vi "ModeMgr.List Modes.vi"(11 "Modes":T1[](array[typedef])=[{"Name"="", "Color"=0, "Options"=[{"Option"="Display Result Data Details", "Level"=0}, {"Option"="Not Reset SN between Tests", "Level"=0}, {"Option"="Not Validate Operator", "Level"=0}, {"Option"="Not Validate SN", "Level"=0}, {"Option"="Disable Results", "Level"=0}, {"Option"="Can Access Station Module", "Level"=0}, {"Option"="Can Edit EQ List", "Level"=0}, {"Option"="Can Clear Warnings", "Level"=0}, {"Option"="Can Clear Errors", "Level"=0}, {"Option"="Can View Config", "Level"=0}, {"Option"="Can Edit Options", "Level"=0}, {"Option"="Can Select Sequence", "Level"=0}, {"Option"="Can Generate Reports", "Level"=0}, {"Option"="Disable Start with SN Entry", "Level"=0}], "Password"=""}, {"Name"="", "Color"=0, "Options"=[{"Option"="Display Result Data Details", "Level"=0}, {"Option"="Not Reset SN between Tests", "Level"=0}, {"Option"="Not Validate Operator", "Level"=0}, {"Option"="Not Validate SN", "Level"=0}, {"Option"="Disable Results", "Level"=0}, {"Option"="Can Access Station Module", "Level"=0}, {"Option"="Can Edit EQ List", "Level"=0}, {"Option"="Can Clear Warnings", "Level"=0}, {"Option"="Can Clear Errors", "Level"=0}, {"Option"="Can View Config", "Level"=0}, {"Option"="Can Edit Options", "Level"=0}, {"Option"="Can Select Sequence", "Level"=0}, {"Option"="Can Generate Reports", "Level"=0}, {"Option"="Disable Start with SN Entry", "Level"=0}], "Password"=""}, {"Name"="", "Color"=0, "Options"=[{"Option"="Display Result Data Details", "Level"=0}, {"Option"="Not Reset SN between Tests", "Level"=0}, {"Option"="Not Validate Operator", "Level"=0}, {"Option"="Not Validate SN", "Level"=0}, {"Option"="Disable Results", "Level"=0}, {"Option"="Can Access Station Module", "Level"=0}, {"Option"="Can Edit EQ List", "Level"=0}, {"Option"="Can Clear Warnings", "Level"=0}, {"Option"="Can Clear Errors", "Level"=0}, {"Option"="Can View Config", "Level"=0}, {"Option"="Can Edit Options", "Level"=0}, {"Option"="Can Select Sequence", "Level"=0}, {"Option"="Can Generate Reports", "Level"=0}, {"Option"="Disable Start with SN Entry", "Level"=0}], "Password"=""}, {"Name"="", "Color"=0, "Options"=[{"Option"="Display Result Data Details", "Level"=0}, {"Option"="Not Reset SN between Tests", "Level"=0}, {"Option"="Not Validate Operator", "Level"=0}, {"Option"="Not Validate SN", "Level"=0}, {"Option"="Disable Results", "Level"=0}, {"Option"="Can Access Station Module", "Level"=0}, {"Option"="Can Edit EQ List", "Level"=0}, {"Option"="Can Clear Warnings", "Level"=0}, {"Option"="Can Clear Errors", "Level"=0}, {"Option"="Can View Config", "Level"=0}, {"Option"="Can Edit Options", "Level"=0}, {"Option"="Can Select Sequence", "Level"=0}, {"Option"="Can Generate Reports", "Level"=0}, {"Option"="Disable Start with SN Entry", "Level"=0}], "Password"=""}] {"Color" items=["Red", "Yellow", "Orange", "Green", "SkyBlue", "Blue", "Purple", "Pink", "Grey"]}) -> (3 "Names":string[](array[string]))   [LabVIEW 2018]
uses:
  ModeMgr.Mode Settings_Config View.ctl
  ModeMgr.Mode Settings.ctl
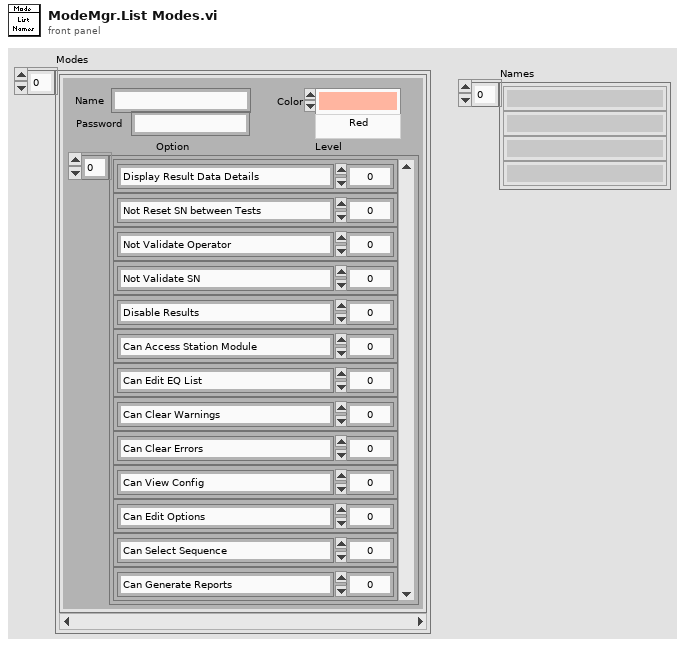
[diagram p1: front panel]
types:
  T1 = typedef "ModeMgr.Mode Settings_Config View.ctl" = cluster{"Name":string, "Color":u16, "Options":T2[], "Password":string}
  T2 = typedef "ModeMgr.Mode Settings.ctl" = cluster{"Option":string, "Level":i32}
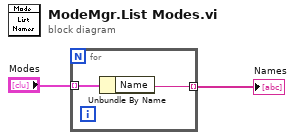
[diagram p0: block diagram]
diagram:
  n1 = for {
    tunnel: "Modes" -> [w4] mode=indexing
    tunnel: [w3] -> w2 mode=indexing
    n2 = Unbundle By Name(w4) -> ("Name"=w3:string)
  }
  "Names" <- w2
